vi "img_data_to_cluster.vi"(8 "error in (no error)":errorcluster, 11 "Input path":path) -> (0 "error out":errorcluster, 2 "Image":T1, 3 "Output path":path)   [LabVIEW 2020]
uses:
  #typedef_cluster_Image.ctl
  #typedef_cluster_Image_Thumbnail.ctl
  <vilib>/vision/Image Controls.llb/IMAQ Image.ctl
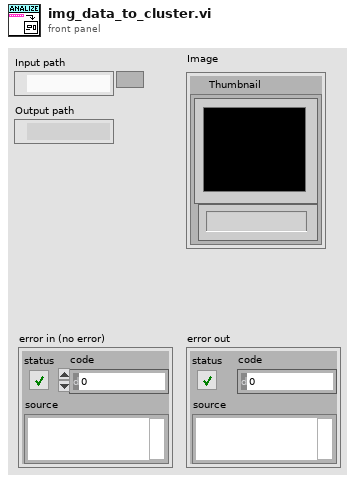
[diagram p1: front panel]
types:
  T1 = typedef "#typedef_cluster_Image.ctl" = cluster{"Thumbnail":T2}
  T2 = typedef "#typedef_cluster_Image_Thumbnail.ctl" = cluster{"Image":T3, "ImageName":string}
  T3 = typedef "IMAQ Image.ctl" = refnum<image>
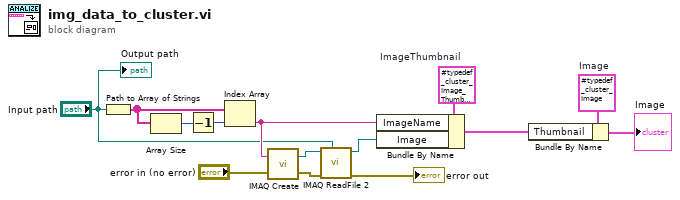
[diagram p0: block diagram]
diagram:
  w10 = T1 {"Thumbnail"={"Image"=refnum, "ImageName"=""}}  # Image
  w14 = T2 {"Image"=refnum, "ImageName"=""}  # ImageThumbnail
  n1 = Path to Array of Strings(0:"Input path") -> (2:w13:string[])  [unwired: 1 out]
  n2 = Array Size(array=w13) -> (size(s)=w12:i32)
  n3 = Decrement(x=w12) -> (x-1=w11:i32)
  n4 = Index Array(array=w13, index=w11) -> (element=w5:string)
  n5 = call "IMAQ Create"("Image Name"=w5, "error in (no error)"="error in (no error)") -> ("New Image"=w7:T3, "error out"=w6:errorcluster)  [unwired: 3 in]
  n6 = call "IMAQ ReadFile 2"("File Path"="Input path", "error in (no error)"=w6, "Image"=w7) -> ("error out"=→"error out":errorcluster, "Image Out"=w3:T3)  [unwired: 4 in, 3 out]
  n7 = Bundle By Name(cluster=w14, "ImageName"=w5, "Image"=w3) -> (w9:T2)
  n8 = Bundle By Name(cluster=w10, "Thumbnail"=w9) -> (→"Image":T1)
  "Output path" <- "Input path"
